vi "Inches_to_Counts.vi"(8 "Encoder Counts Input":dbl, 11 "Inches":dbl) -> (0 "Inches Output":dbl, 3 "Encoder Counts":i64)   [LabVIEW 2020]
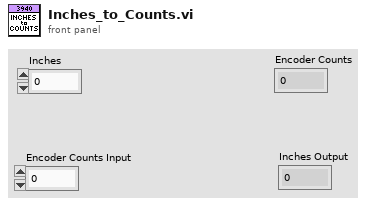
[diagram p1: front panel]
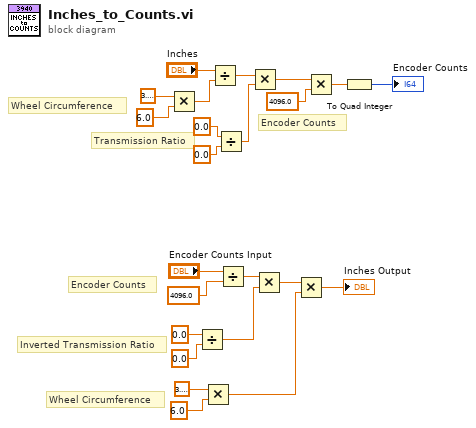
[diagram p0: block diagram]
diagram:
  # "Wheel Circumference"
  # "Inverted Transmission Ratio"
  # "Encoder Counts"
  # "Encoder Counts"
  # "Transmission Ratio"
  # "Wheel Circumference"
  n1 = Multiply(x=3.141592653589793, y=6.0) -> (x*y=w20:dbl)
  n2 = Divide(x=0.0, y=0.0) -> (x/y=w8:dbl)
  n3 = Multiply(x=3.141592653589793, y=6.0) -> (x*y=w2:dbl)
  n4 = Divide(x="Inches", y=w20) -> (x/y=w19:dbl)
  n5 = Divide(x=0.0, y=0.0) -> (x/y=w16:dbl)
  n6 = Divide(x="Encoder Counts Input", y=4096.0) -> (x/y=w9:dbl)
  n7 = Multiply(x=w19, y=w16) -> (x*y=w15:dbl)
  n8 = Multiply(x=w9, y=w8) -> (x*y=w5:dbl)
  n9 = Multiply(x=w5, y=w2) -> (x*y=→"Inches Output":dbl)
  n10 = Multiply(x=w15, y=4096.0) -> (x*y=w13:dbl)
  n11 = To Quad Integer(1:w13) -> (0:→"Encoder Counts":i64)
